vi "Actor Core.vi"(8 "error in":errorcluster, 11 "RDS Logger Actor in":refnum<class "RDS Logger Actor.lvclass">) -> (0 "error out":errorcluster, 3 "Actor out":refnum<class "Actor.lvclass">)   [LabVIEW 2015, in "RDS Logger Actor.lvlib" / "RDS Logger Actor.lvclass"]
doc: "(<B>Filename</B>: Actor Framework.lvlib:Actor.lvclass:Actor Core.vi)\n\nReceives messages to the actor, reacts to them, and initiates any error handling that may shut the actor down.\n\nDescendant classes may override this VI to append parallel tasks for the actor to complete while it handles messages. Overrides use the Call Parent Method node."
uses:
  RDS Logger Actor.lvclass
  RDS Parent Actor/RDS Parent Actor/RDS Parent Actor.lvclass
  <vilib>/ActorFramework/Actor/Actor.lvclass
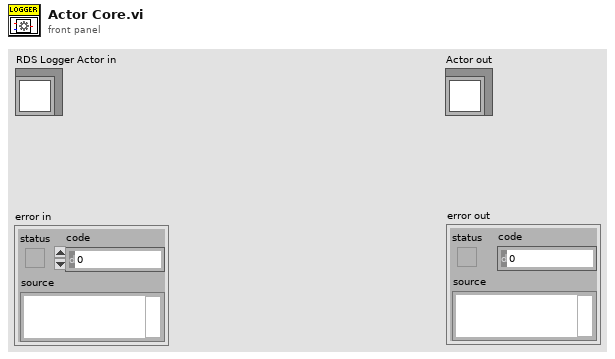
[diagram p1: front panel]
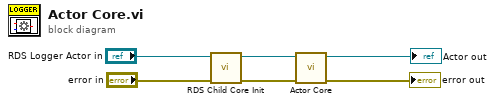
[diagram p0: block diagram]
diagram:
  n1 = call "RDS Child Core Init.vi"("error in (no error)"="error in", "RDS Parent Actor in"="RDS Logger Actor in") -> ("error out"=w1:errorcluster, "RDS Parent Actor out"=w3:refnum<class "RDS Logger Actor.lvclass">)  [unwired: 6 in, 2 out]
  n2 = call-parent "Actor Core.vi"("error in"=w1, "Actor in"=w3) -> ("error out"=→"error out":errorcluster, "Actor out"=→"Actor out":refnum<class "Actor.lvclass">)  [unwired: 8 in]
